vi "Tag To BFS Index.vi"(10 "Tag In":string, 11 "Root Tag":string) -> (2 "BFS Index Out":i32[](array[numeric]))   [LabVIEW 2024]
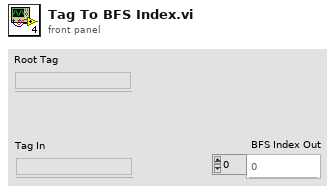
[diagram p1: front panel]
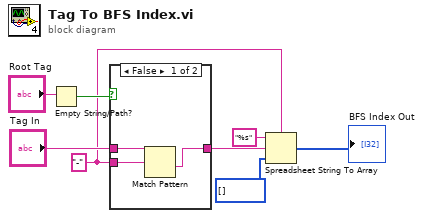
[diagram p0: block diagram]
diagram:
  w1 = "-" ("delimiter (Tab)")
  n1 = Empty String/Path?(string/path="Root Tag") -> (empty?=w4:bool)
  n2 = case shown="False" w4 {
    tunnel: "Tag In" -> [w11 w12]
    tunnel: [w10 w12] -> w2
    tunnel: w1 -> [w9 _]
    frame False {
      n3 = Match Pattern(string=w11, regular expression=w9) -> (after substring=w10:string)  [unwired: 1 in, 3 out]
    }
    frame True {
    }
  }
  n4 = Spreadsheet String To Array(delimiter (Tab)=w1, format string="%s", spreadsheet string=w2, array type (2D Dbl)=i32[] []) -> (array=→"BFS Index Out":i32[])
